vi "setFPGAReference.vi"(10 "FPGAReference":refnum<k20>, 11 "MyHealthAndStatusReadFIFO in":refnum<class "ModbusPort1TimestampFIFO.lvclass">) -> (3 "MyHealthAndStatusReadFIFO out":refnum<class "ModbusPort1TimestampFIFO.lvclass">)   [LabVIEW 2016, in "ModbusPort1TimestampFIFO.lvclass"]
uses:
  ModbusPort1TimestampFIFO.lvclass
  ModbusPort1TimestampFIFO.lvclass/ModbusPort1TimestampFIFO.ctl
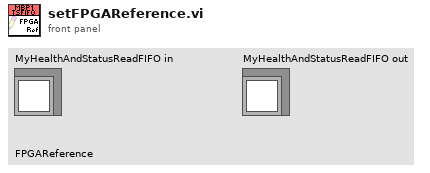
[diagram p1: front panel]
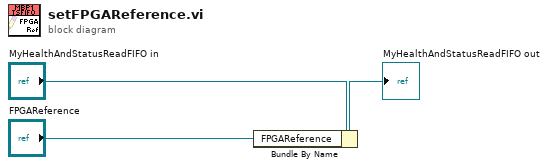
[diagram p0: block diagram]
diagram:
  n1 = Bundle By Name(cluster="MyHealthAndStatusReadFIFO in", "FPGAReference"="FPGAReference") -> (→"MyHealthAndStatusReadFIFO out":refnum<class "ModbusPort1TimestampFIFO.lvclass">)
